vi "Zaber A Series IOs.vi"() -> ()   [LabVIEW 2013]
doc: "This example shows how you can query and set the IOs of the A-MCB2 controller."
uses:
  Zaber A Series.lvlib
panel:
  out "Digital Output 4":bool
  out "Digital Output 3":bool
  out "Digital Output 2":bool
  out "Digital Output 1":bool
  out "Analog In 4 (Volts)":string
  out "Analog In 3 (Volts)":string
  out "Analog In 2 (Volts)":string
  out "Analog In 1 (Volts)":string
  out "Digital In 4":bool
  out "Digital In 3":bool
  out "Digital In 2":bool
  out "Digital In 1":bool
  in  "Digital Out 4":bool
  in  "Digital Out 3":bool
  in  "Digital Out 2":bool
  in  "Digital Out 1":bool
  in  "VISA resource name":refnum<visa-resource-name>
  out "Port Open":bool
  in  "Quit":bool
  in  "Open Port":bool
  in  "Close Port":bool
  # "(c) 2014 Zaber Technologies.  ALL RIGHTS RESERVED."
  # "The A-MCB2 controller has inputs and outputs. This example shows how you can read and parse these inputs. Once the port is open, it will poll the IOs and update the information. You can easily switch the digital outputs to update them as well. \n\nAdditionally this example uses a persistent interface so you can manage the port while the VI is running. This can be used as a template for similar programs (the Front Panel example also uses this template). \n\nNote: This example will only function with the A-MCB2 controller, and also the Quit button takes a little while to complete."
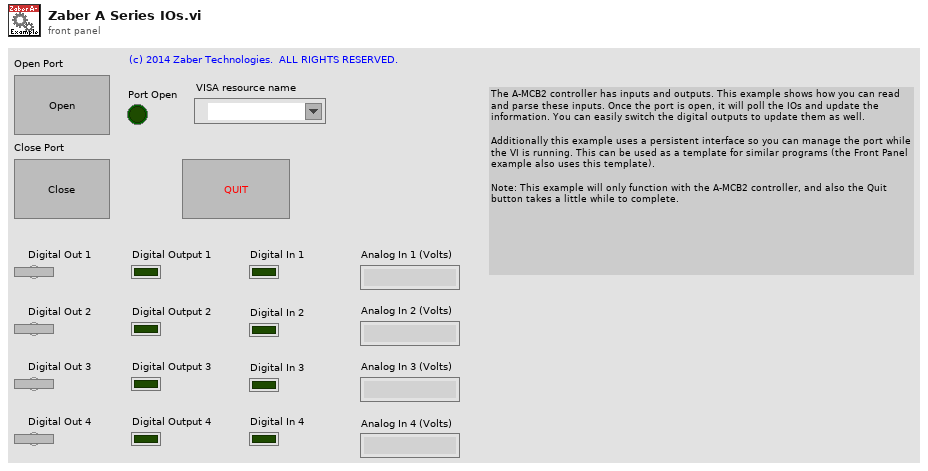
[diagram p1: front panel]
types:
  T1 = cluster{"Device":string, "Axis":string, "Reply Flag":string, "Status":string, "Warning Flags":string, "Data":string}[]
  T2 = cluster{"Device":string, "Axis":string, "Reply Flag":string, "Status":string, "Warning Flags":string, "Data":string}
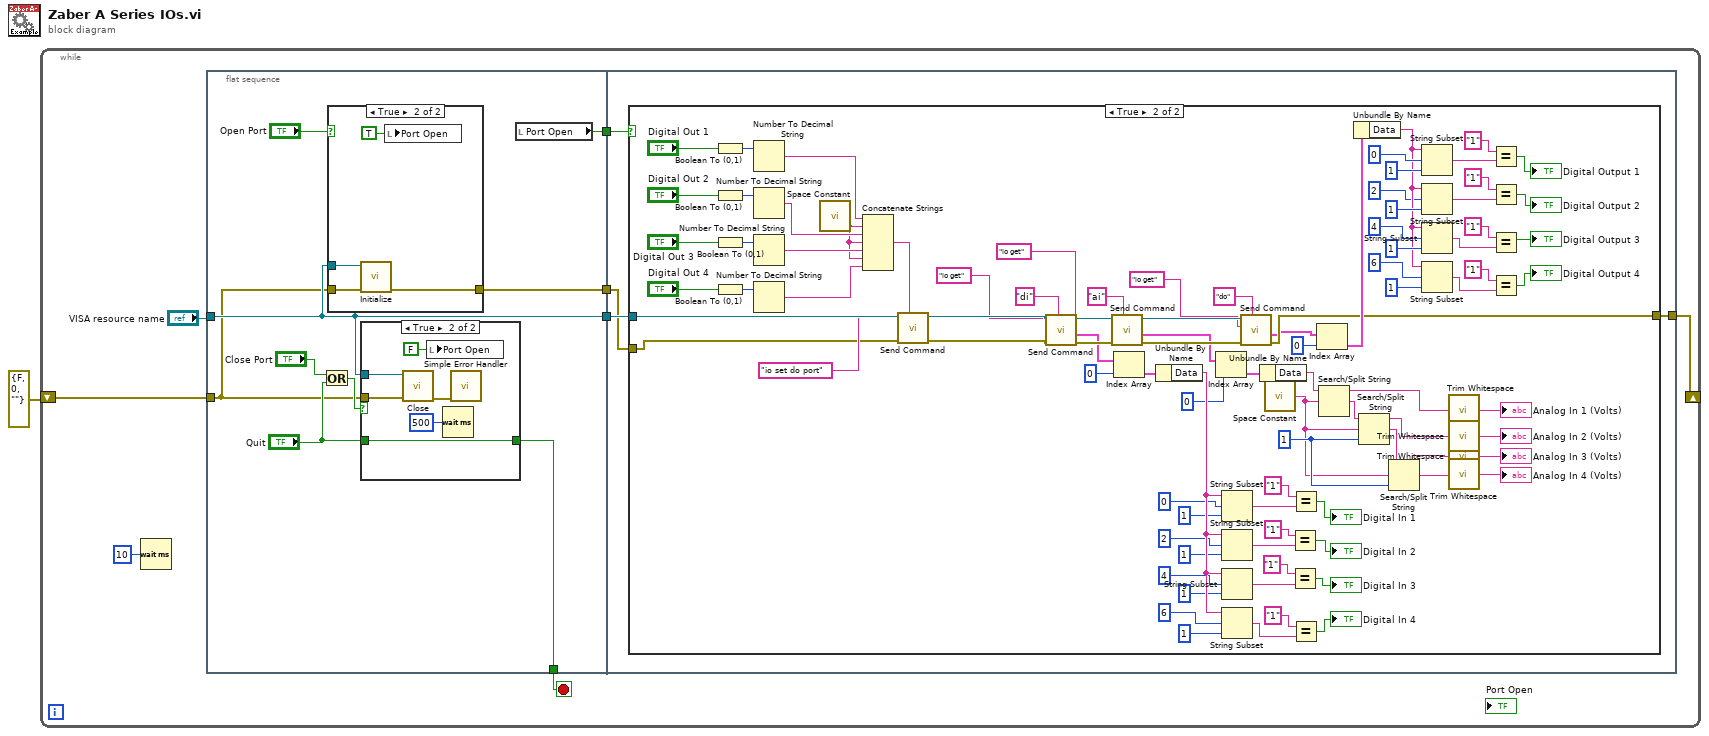
[diagram p0: block diagram]
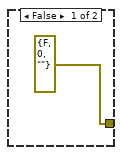
[diagram p3: hidden frame]
diagram:
  n1 = while {
    shift-right: [w4] -> _
    shift-left: errorcluster {"status"=FALSE, "code"=0, "source"=""} ("error out") -> [w3]
    stop <- w7 stop-if-true
    n2 = Wait (ms)(milliseconds to wait=u32 10) -> ()  [unwired: 1 out]
    n3 = flat-sequence {
      tunnel: "VISA resource name" -> [w14]
      tunnel: [w14] -> w9
      tunnel: [w13] -> w8
      tunnel: [w12] -> w7
      tunnel: [w11] -> w5
      tunnel: w3 -> [w10]
      tunnel: w9 -> [w33]
      tunnel: w8 -> [w34]
      tunnel: w5 -> [w32]
      tunnel: [w31] -> w4
      frame #0 {
        n4 = Or(x="Close Port", y="Quit") -> (x .or. y?=w17:bool)
        n5 = case shown="True" "Open Port" {
          tunnel: w14 -> [_ w30]
          tunnel: [errorcluster {"status"=FALSE, "code"=0, "source"=""} ("error in (no error)") w28] -> w11
          tunnel: w10 -> [_ w27]
          frame False {
          }
          frame True {
            n6 = call "Initialize.vi"("error in (no error)"=w27, "VISA resource name"=w30) -> ("error out"=w28:errorcluster)  [unwired: 8 in, 1 out]
            n7 = local write "Port Open"(TRUE) -> ()
          }
        }
        n8 = case shown="True" w17 {
          tunnel: w14 -> [_ w23]
          tunnel: [w19 w25] -> w12
          tunnel: "Quit" -> [w19 w25]
          tunnel: w10 -> [_ w22]
          frame False {
          }
          frame True {
            n9 = call "Close.vi"("error in (no error)"=w22, "VISA resource name"=w23) -> ("error out"=w21:errorcluster)  [unwired: 9 in]
            n10 = local write "Port Open"(FALSE) -> ()
            n11 = Wait (ms)(milliseconds to wait=u32 500) -> ()  [unwired: 1 out]
            n12 = call <vilib>:"Simple Error Handler.vi"("error in (no error)"=w21) -> ()  [unwired: 4 in, 5 out]
          }
        }
        n13 = local read "Port Open"() -> (w13:bool)
      }
      frame #1 {
        n14 = case shown="True" w34 {
          tunnel: w33 -> [_ w55]
          tunnel: w32 -> [w35 w53]
          tunnel: [w35 w42] -> w31
          frame False {
          }
          frame True {
            w69 = 1 ("offset (0)")
            n15 = Boolean To (0,1)(Boolean="Digital Out 1") -> (0, 1=w124:i16)
            n16 = Boolean To (0,1)(Boolean="Digital Out 2") -> (0, 1=w123:i16)
            n17 = Boolean To (0,1)(Boolean="Digital Out 3") -> (0, 1=w122:i16)
            n18 = Boolean To (0,1)(Boolean="Digital Out 4") -> (0, 1=w121:i16)
            n19 = Number To Decimal String(number=w124) -> (decimal integer string=w117:string)  [unwired: 1 in]
            n20 = Number To Decimal String(number=w123) -> (decimal integer string=w116:string)  [unwired: 1 in]
            n21 = Number To Decimal String(number=w122) -> (decimal integer string=w115:string)  [unwired: 1 in]
            n22 = Number To Decimal String(number=w121) -> (decimal integer string=w114:string)  [unwired: 1 in]
            n23 = call <vilib>:"Space Constant.vi"() -> ("String"=w113:string)
            n24 = Concatenate Strings(w117, w113, w116, w113, w115, w113, w114) -> (w52:string)
            n25 = call "Send Command.vi"("Data"=w52, "error in (no error)"=w53, "Command"="io set do port" ("Complete Command List"), "VISA resource name"=w55) -> ("error out"=w50:errorcluster, "VISA resource name out"=w51:refnum<visa-resource-name>)  [unwired: 3 in, 3 out]
            n26 = call "Send Command.vi"("Data"="di", "error in (no error)"=w50, "Command"="io get" ("Complete Command List"), "VISA resource name"=w51) -> ("error out"=w48:errorcluster, "Response Bundle Array"=w46:T1, "VISA resource name out"=w44:refnum<visa-resource-name>)  [unwired: 3 in, 2 out]
            n27 = call "Send Command.vi"("Data"="ai", "error in (no error)"=w48, "Command"="io get" ("Complete Command List"), "VISA resource name"=w44) -> ("error out"=w47:errorcluster, "Response Bundle Array"=w38:T1, "VISA resource name out"=w43:refnum<visa-resource-name>)  [unwired: 3 in, 2 out]
            n28 = Index Array(array=w46, index=0 ("index (row)")) -> (element=w128:T2)
            n29 = Unbundle By Name(w128) -> ("Data"=w100:string)
            n30 = Index Array(array=w38, index=0 ("index (row)")) -> (element=w127:T2)
            n31 = String Subset(string=w100, offset (0)=0, length (rest)=1 ("length (rest)")) -> (substring=w111:string)
            n32 = String Subset(string=w100, offset (0)=2, length (rest)=1 ("length (rest)")) -> (substring=w106:string)
            n33 = String Subset(string=w100, offset (0)=4, length (rest)=1 ("length (rest)")) -> (substring=w104:string)
            n34 = String Subset(string=w100, offset (0)=6, length (rest)=1 ("length (rest)")) -> (substring=w102:string)
            n35 = call "Send Command.vi"("Data"="do", "error in (no error)"=w47, "Command"="io get" ("Complete Command List"), "VISA resource name"=w43) -> ("error out"=w42:errorcluster, "Response Bundle Array"=w41:T1)  [unwired: 3 in, 3 out]
            n36 = Unbundle By Name(w127) -> ("Data"=w72:string)
            n37 = call <vilib>:"Space Constant.vi"() -> ("String"=w68:string)
            n38 = Equal?(x="1", y=w106) -> (x = y?=→"Digital In 2":bool)
            n39 = Equal?(x="1", y=w104) -> (x = y?=→"Digital In 3":bool)
            n40 = Equal?(x="1", y=w111) -> (x = y?=→"Digital In 1":bool)
            n41 = Equal?(x="1", y=w102) -> (x = y?=→"Digital In 4":bool)
            n42 = Index Array(array=w41, index=0 ("index (row)")) -> (element=w126:T2)
            n43 = Search/Split String(string=w72, search string/char (-)=w68) -> (substring before match=w64:string, match + rest of string=w71:string)  [unwired: 1 in, 1 out]
            n44 = Unbundle By Name(w126) -> ("Data"=w59:string)
            n45 = Search/Split String(string=w71, search string/char (-)=w68, offset (0)=w69) -> (substring before match=w66:string, match + rest of string=w70:string)  [unwired: 1 out]
            n46 = Search/Split String(string=w70, search string/char (-)=w68, offset (0)=w69) -> (substring before match=w62:string, match + rest of string=w67:string)  [unwired: 1 out]
            n47 = String Subset(string=w59, offset (0)=0, length (rest)=1 ("length (rest)")) -> (substring=w90:string)
            n48 = String Subset(string=w59, offset (0)=2, length (rest)=1 ("length (rest)")) -> (substring=w85:string)
            n49 = String Subset(string=w59, offset (0)=4, length (rest)=1 ("length (rest)")) -> (substring=w83:string)
            n50 = String Subset(string=w59, offset (0)=6, length (rest)=1 ("length (rest)")) -> (substring=w81:string)
            n51 = call <vilib>:"Trim Whitespace.vi"("string"=w64) -> ("trimmed string"=→"Analog In 1 (Volts)":string)  [unwired: 1 in]
            n52 = call <vilib>:"Trim Whitespace.vi"("string"=w66) -> ("trimmed string"=→"Analog In 2 (Volts)":string)  [unwired: 1 in]
            n53 = call <vilib>:"Trim Whitespace.vi"("string"=w62) -> ("trimmed string"=→"Analog In 3 (Volts)":string)  [unwired: 1 in]
            n54 = call <vilib>:"Trim Whitespace.vi"("string"=w67) -> ("trimmed string"=→"Analog In 4 (Volts)":string)  [unwired: 1 in]
            n55 = Equal?(x="1", y=w90) -> (x = y?=→"Digital Output 1":bool)
            n56 = Equal?(x="1", y=w85) -> (x = y?=→"Digital Output 2":bool)
            n57 = Equal?(x="1", y=w83) -> (x = y?=→"Digital Output 3":bool)
            n58 = Equal?(x="1", y=w81) -> (x = y?=→"Digital Output 4":bool)
          }
        }
      }
    }
  }
